vi "Demo Math Tester.vi"() -> ()   [LabVIEW 2014]
uses:
  <vilib>/Utility/miscctls.llb/LVRowAndColumnTypeDef.ctl
  <vilib>/Utility/miscctls.llb/LVPointTypeDef.ctl
  MathLoop/TypeDefs/ParsedExpression.ctl
  MathLoop/TypeDefs/typeMed.ctl
  MathLoop/TypeDefs/Conf. Gral.ctl
  APIs/Data Queue/Acquisition Data 1 Sample Cluster.ctl
  <vilib>/Analysis/2dsp.llb/Real FFT.vi
  <vilib>/Analysis/2dsp.llb/Inverse Real FFT.vi
  <vilib>/Analysis/2dsp.llb/Inverse Complex FFT.vi
  MathLoop/TypeDefs/Globals.vi
  APIs/Message Queue/Enqueue Message (Single).vi
  <vilib>/Utility/file.llb/Write To Spreadsheet File (string).vi
  APIs/Data Queue/WINFAS 2 Data Queue.lvlib
  APIs/Message Queue/WINFAS 2 Message Queue.lvlib
  MathLoop/MathLoop.lvlib
  <vilib>/Analysis/NI_AALPro.lvlib
panel:
  in  "Config:Mapp":bool
  out "MedPath":string
  out "TransPath":string caption="Último Cálculo:"
  in  "error in (no error)":errorcluster
  out "Time":dbl=0.7666387252129425 format="%#_6fseg"
  out "LAST":string="28/08/2015 08:45:35 a.m." caption="Último Cálculo:"
  in  "Medicion (Solo P/ Resultado Post-Proceso):":i32=1 min=0 max=0 format="M%.0f"
  out "Medición":string[][](table)
  out "Curva de Engranes":dbl[][](graph)
  out "Transductores":string[][](table)
  in  "Config Aux & Med":bool
  in  "Save Cfg":bool
  in  "Start":bool
  in  "Open Cfg":bool
  in  "New Cfg":bool
  # "Configuración"
  # "Curva de Engrane"
  # "Archivos:"
  # "Tabla de Transductores"
  # "Proceso de medición"
  # "Último Cálculo:"
  # "Tiempo de Cálculo:"
  # "Medición"
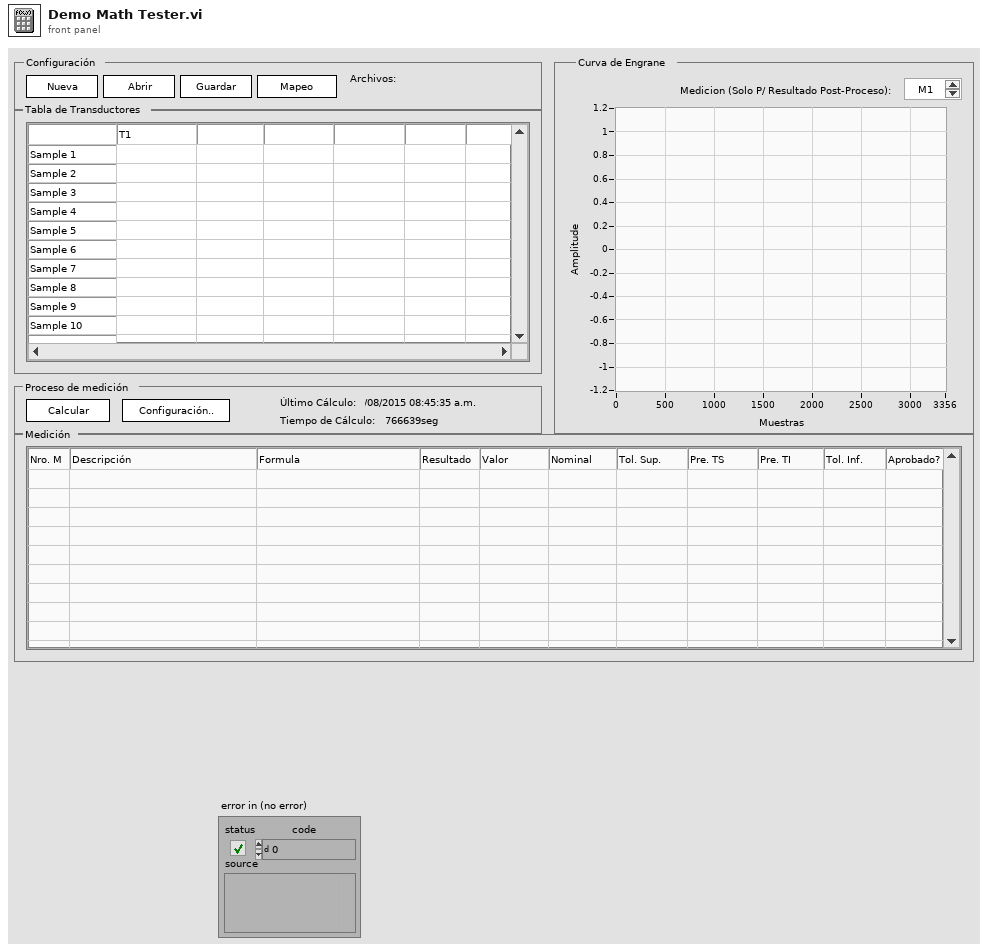
[diagram p1: front panel]
types:
  T1 = typedef "MathLoop.lvlib/ParsedExpression.ctl" = cluster{"RPN ":string[], "Constantes":sgl[], "Variables":string[], "Formula":string, "Tipo de Med":T2, "Med?":bool, "Descripción":string, "Nominal":sgl, "Tol Sup":sgl, "Pre TS":sgl, "Pre TI":sgl, "Tol Inf":sgl}
  T2 = typedef "MathLoop.lvlib/typeMed.ctl" = string
  T3 = typedef "MathLoop.lvlib/Conf. Gral.ctl" = cluster{"Engranometro":cluster{"Cant. Dientes x pieza":i32, "Nro. Dientes (Frp)":i32, "Armonicas":i32}}
  T4 = cluster{"Variable Data Out":cluster{"Kcte":sgl[], "Dcte":sgl[], "Aux":sgl[][], "Transductores":sgl[][]}, "Array":sgl[], T1[], "Array Med":sgl[][], "Conf. General":T3}
  T5 = typedef "LVPointTypeDef.ctl" = cluster{"Horizontal":i16, "Vertical":i16}
  T6 = typedef "LVRowAndColumnTypeDef.ctl" = cluster{"Row":i32, "Column":i32}
  T7 = enum32{"invalid app kind", "Development System", "Run Time System", "Student Edition", "Embedded LabVIEW", "Evaluation", "Custom"}
  T8 = typedef "WINFAS 2 Message Queue.lvlib/All Message Queues.ctl" = cluster{"CORE":refnum<queue>, "Event UI":refnum<queue>, "Display UI":refnum<queue>, "MATH":refnum<queue>, "SEQ":refnum<queue>, "DB":refnum<queue>, "ERR":refnum<queue>, "HAL":refnum<queue>, "HWSync1":refnum<queue>, "HWSync2":refnum<queue>, "HWSync3":refnum<queue>, "HWSync4":refnum<queue>, "HWSync5":refnum<queue>, "HWAsync1":refnum<queue>, "HWAsync2":refnum<queue>, "HWAsync3":refnum<queue>, "HWAsync4":refnum<queue>, "HWAsync5":refnum<queue>, "HWAsync6":refnum<queue>, "HWAsync7":refnum<queue>, "HWAsync8":refnum<queue>, "HWAsync9":refnum<queue>, "HWAsync10":refnum<queue>}
  T9 = typedef "WINFAS 2 Data Queue.lvlib/All Data Queues Cluster.ctl" = cluster{"Queues":cluster{"ACQ HWSync1":refnum<queue>, "ACQ HWSync2":refnum<queue>, "ACQ HWSync3":refnum<queue>, "ACQ HWSync4":refnum<queue>, "ACQ HWSync5":refnum<queue>}, "Notifiers":cluster{"Control":cluster{"CTRL HWSync1":refnum<notifier>, "CTRL HWSync2":refnum<notifier>, "CTRL HWSync3":refnum<notifier>, "CTRL HWSync4":refnum<notifier>, "CTRL HWSync5":refnum<notifier>}, "Acquisition":cluster{"ACQ HWSync1":refnum<notifier>, "ACQ HWSync2":refnum<notifier>, "ACQ HWSync3":refnum<notifier>, "ACQ HWSync4":refnum<notifier>, "ACQ HWSync5":refnum<notifier>}, "Async":cluster{"ACQ HWAsync1":refnum<notifier>, "ACQ HWAsync2":refnum<notifier>, "ACQ HWAsync3":refnum<notifier>, "ACQ HWAsync4":refnum<notifier>, "ACQ HWAsync5":refnum<notifier>, "ACQ HWAsync6":refnum<notifier>, "ACQ HWAsync7":refnum<notifier>, "ACQ HWAsync8":refnum<notifier>, "ACQ HWAsync9":refnum<notifier>, "ACQ HWAsync10":refnum<notifier>}}}
  T10 = cluster{"Array Parsed Expression":T1[], "Nominal":sgl[], "Total Inferior":sgl[], "Total Superior":sgl[], "Pre Total Inferior":sgl[], "Pre Total Superior":sgl[], "Descripción":string[]}
  T11 = typedef "WINFAS 2 Data Queue.lvlib/Acquisition Data 1 Sample Cluster.ctl" = cluster{"TDX":sgl[], "Encoder":sgl}
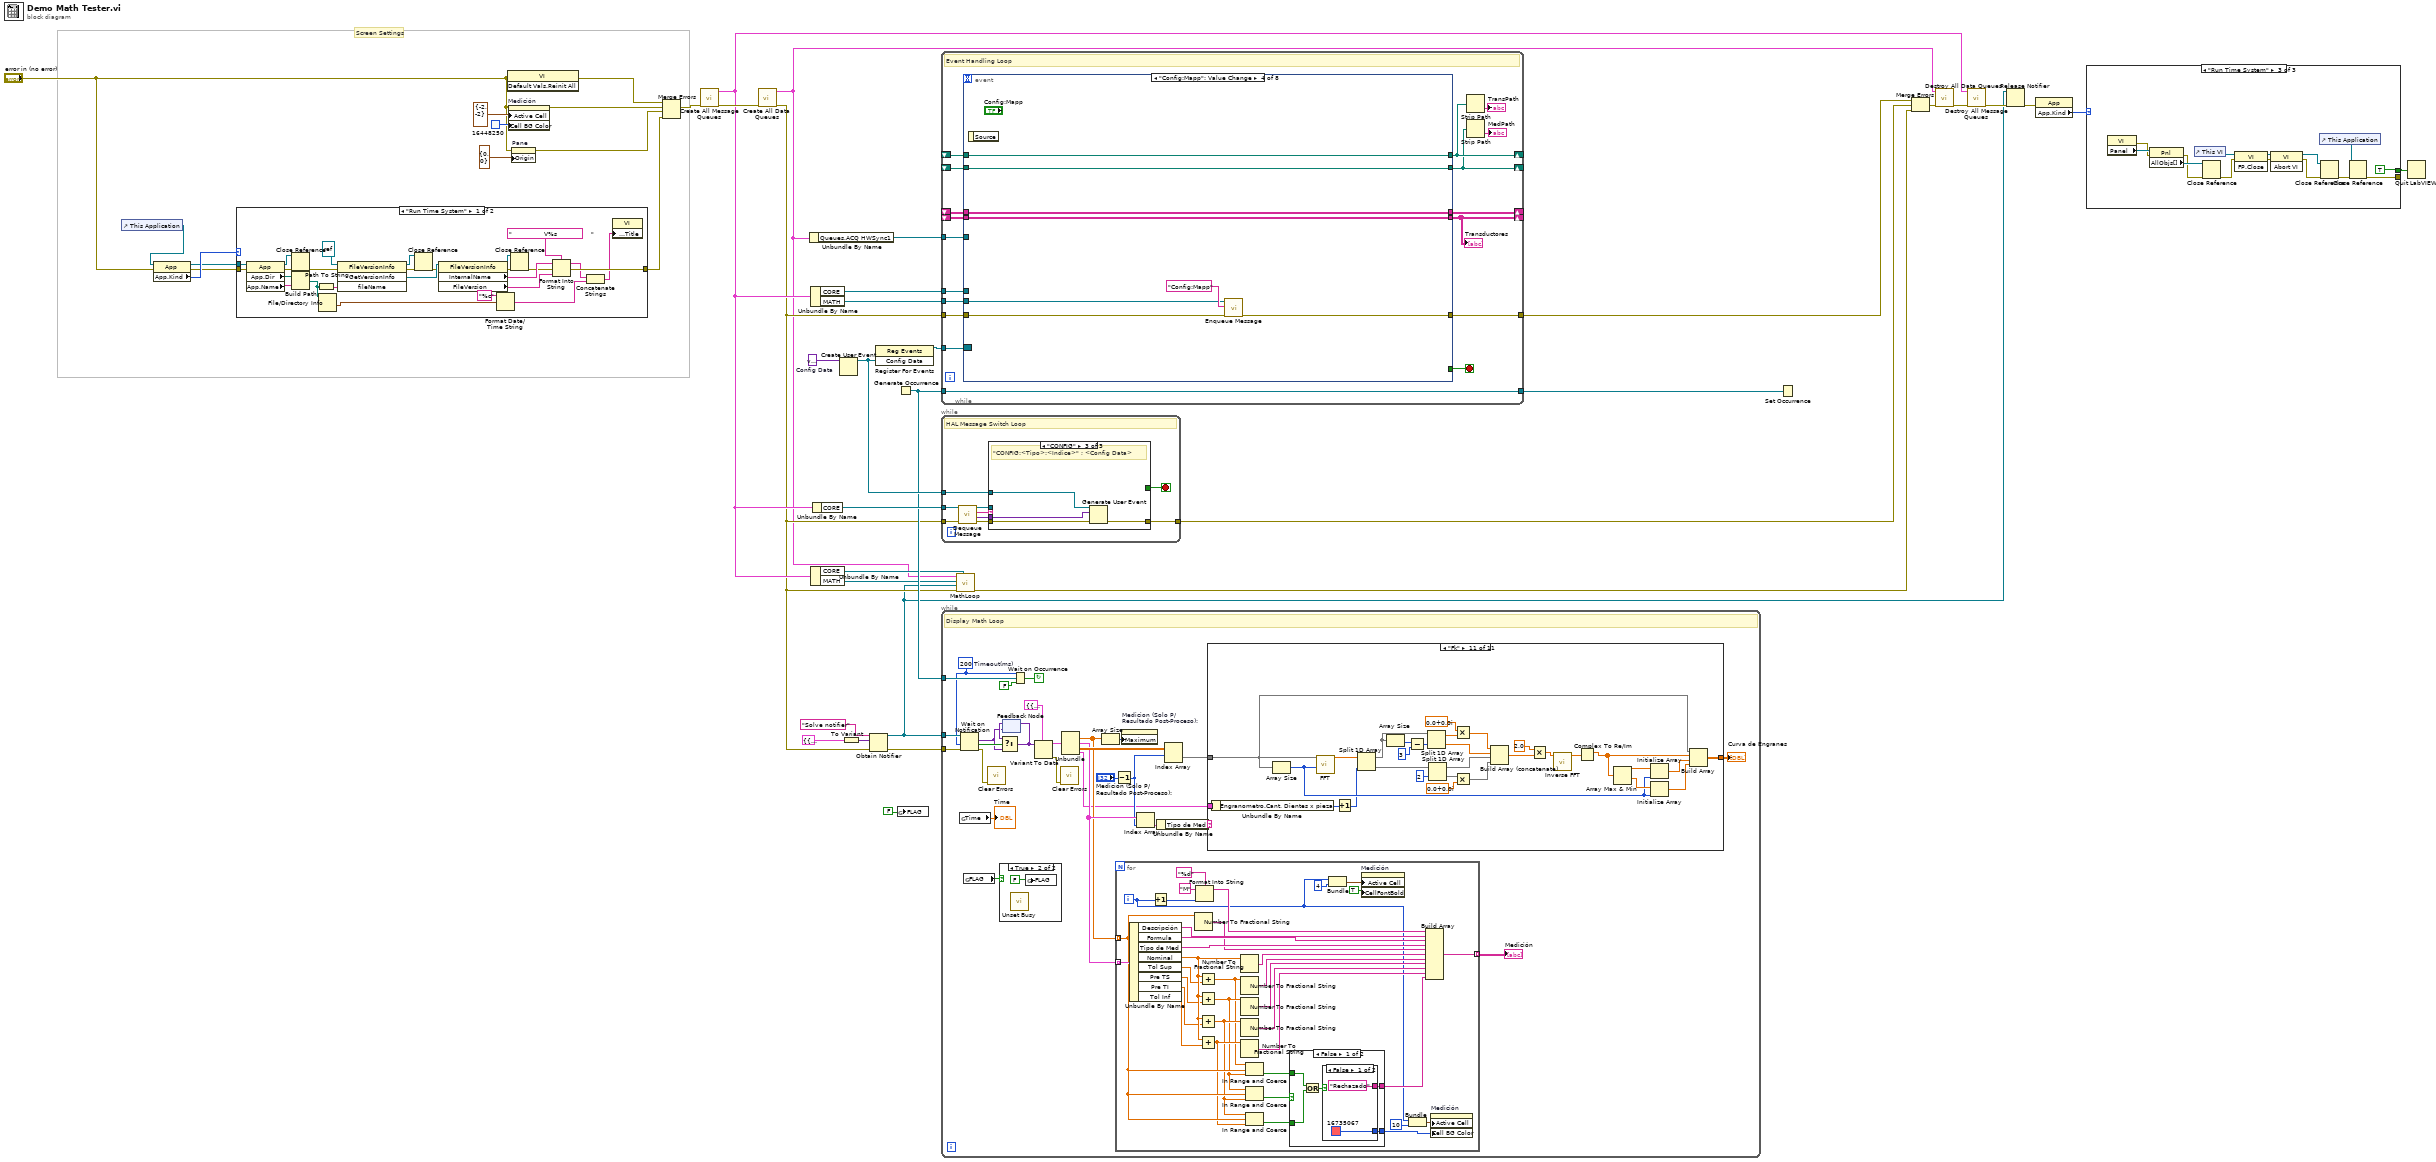
[diagram p0: block diagram]
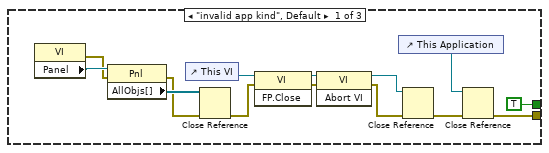
[diagram p3: hidden frame]
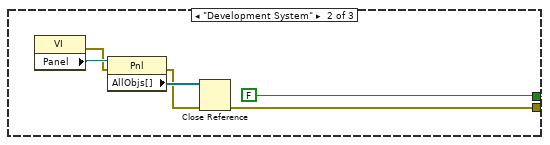
[diagram p4: hidden frame]
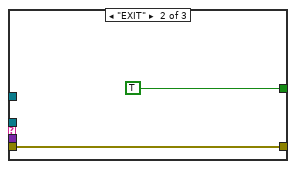
[diagram p6: hidden frame]
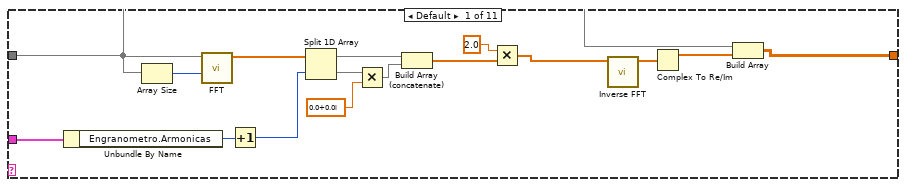
[diagram p8: hidden frame]
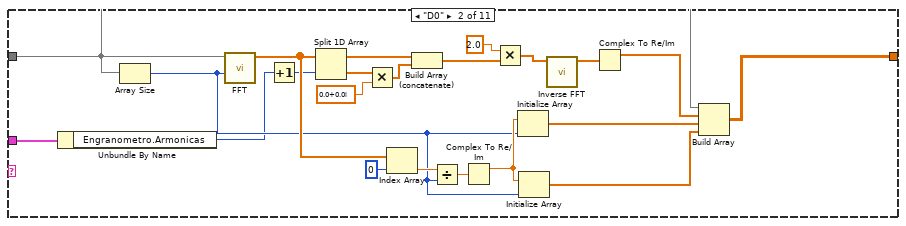
[diagram p9: hidden frame]
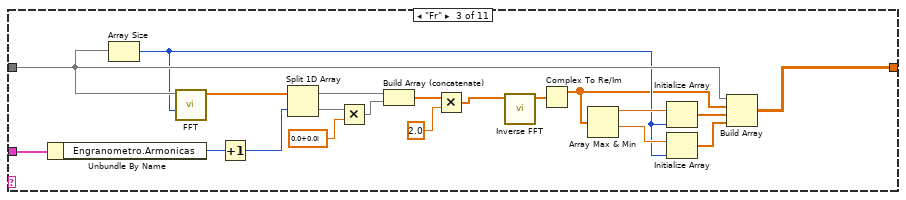
[diagram p10: hidden frame]
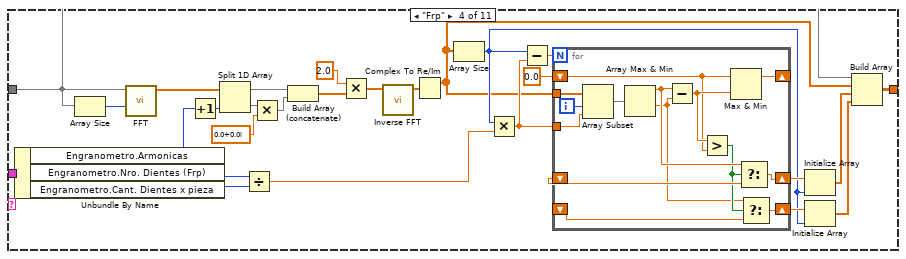
[diagram p11: hidden frame]
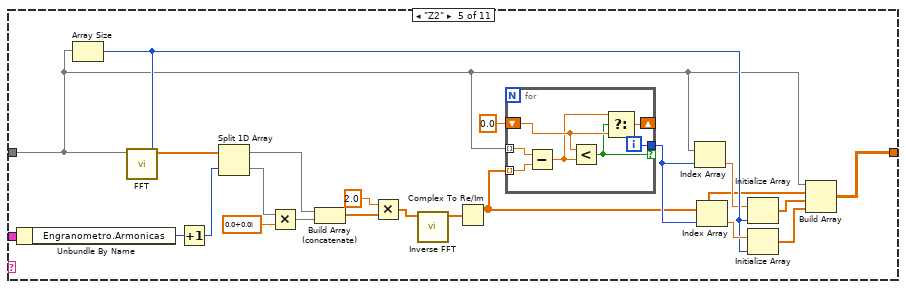
[diagram p12: hidden frame]
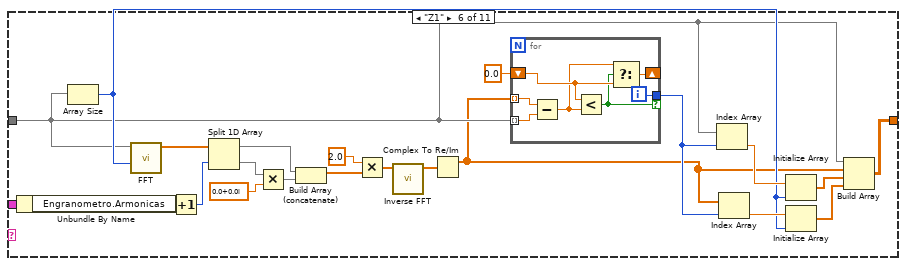
[diagram p13: hidden frame]
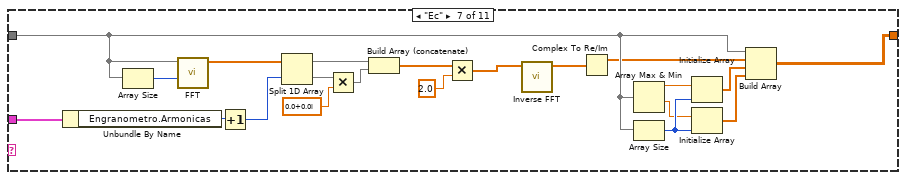
[diagram p14: hidden frame]
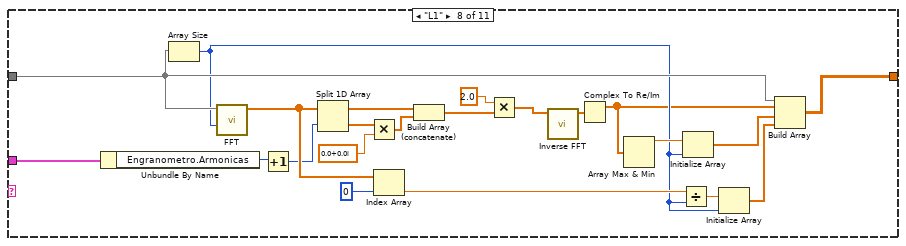
[diagram p15: hidden frame]
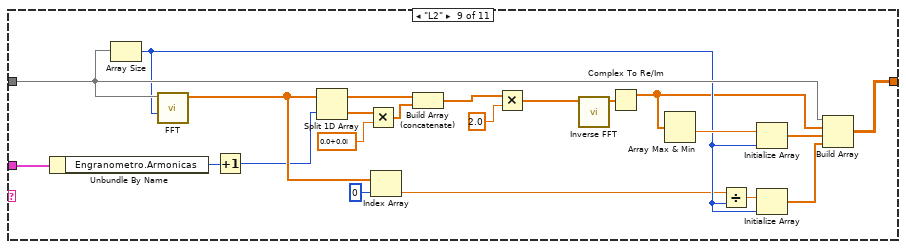
[diagram p16: hidden frame]
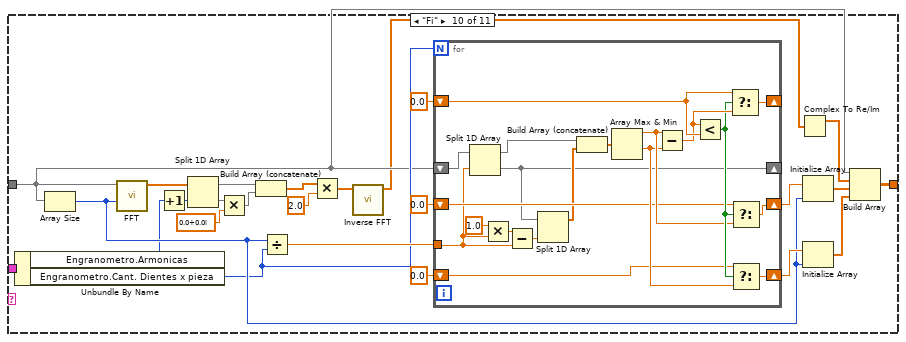
[diagram p17: hidden frame]
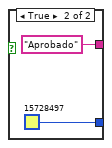
[diagram p18: hidden frame]
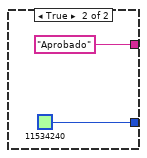
[diagram p19: hidden frame]
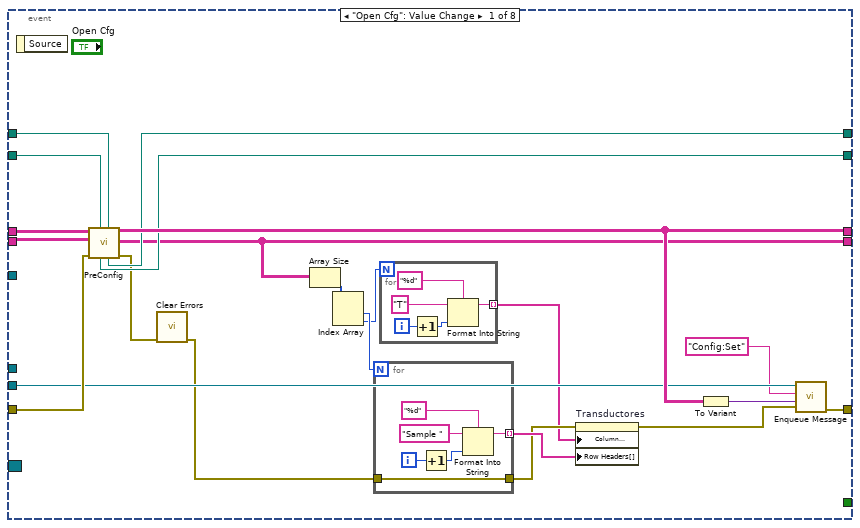
[diagram p20: hidden frame]
diagram:
  w31 = variant  # Config Data
  # "Screen Settings"
  n1 = control-ref of="This Application"() -> (w3:refnum<vi>)
  n2 = property class="App"(reference=w3, error in="error in (no error)") -> (reference out=w4:refnum<vi>, error out=w5:errorcluster, "App.Kind"=w6:T7)
  n3 = case shown="\"Run Time System\"" w6 {
    tunnel: w5 -> [w67 w69]
    tunnel: w4 -> [w68 _]
    tunnel: [w60 w69] -> w1
    frame "Run Time System" {
      n4 = property class="App"(reference=w68, error in=w67) -> (reference out=w48:refnum<vi>, error out=w65:errorcluster, "App.Dir"=w55:path, "App.Name"=w54:string)
      n5 = Close Reference(reference=w48, error in (no error)=w65) -> (error out=w64:errorcluster)
      n6 = Build Path(base path=w55, name or relative path=w54) -> (appended path=w52:path)
      n7 = Path To String(path=w52) -> (string=w66:string)
      n8 = File/Directory Info(path=w52) -> (last mod=w47:timestamp)  [unwired: 1 in, 6 out]
      n9 = invoke class="FileVersionInfo" method="GetVersionInfo"(reference=refnum<k24> refnum, error in=w64, "fileName"=w66) -> (reference out=w50:refnum<k24>, error out=w51:errorcluster, "GetVersionInfo"=w63:refnum<k24>)  [unwired: 1 in, 1 out]
      n10 = Close Reference(reference=w50, error in (no error)=w51) -> (error out=w49:errorcluster)
      n11 = property class="FileVersionInfo"(reference=w63, error in=w49) -> (reference out=w56:refnum<k24>, error out=w58:errorcluster, "InternalName"=w62:string, "FileVersion"=w61:string)
      n12 = Format Date/Time String(time format string (%c)="%c", seconds (now)=w47) -> (date/time string=w45:string)  [unwired: 1 in]
      n13 = Close Reference(reference=w56, error in (no error)=w58) -> (error out=w57:errorcluster)
      n14 = Format Into String(format string="                V%s                 ", initial string=w62, error in=w57, w61) -> (resulting string=w44:string, error out=w60:errorcluster)
      n15 = Concatenate Strings(w44, w45) -> (w43:string)
      n16 = property class="VI"("Front Panel.Title"=w43) -> ()  [unwired: 2 in, 2 out]
    }
    frame "Development System", Default {
    }
  }
  n17 = invoke on="Invoke Node" class="VI" method="Default Vals.Reinit All"(error in="error in (no error)") -> (error out=w18:errorcluster)  [unwired: 2 in, 2 out]
  n18 = property on="Medición" class="Tbl (strict)"(error in="error in (no error)", "Active Cell"=T6 {"Row"=-2, "Column"=-2} ("Active Cell:Active Cell"), "Cell BG Color"=u32 16448250) -> (error out=w19:errorcluster)  [unwired: 1 in, 1 out]
  n19 = property on="Pane" class="Pane"(error in="error in (no error)", "Origin"=T5 {"Horizontal"=0, "Vertical"=0}) -> (error out=w15:errorcluster)  [unwired: 1 in, 1 out]
  n20 = Merge Errors(w18, w19, w15, w1) -> (w20:errorcluster)
  n21 = call "Create All Message Queues.vi"("error in (no error)"=w20) -> ("error out"=w41:errorcluster, "Message Queues Out"=w33:T8)  [unwired: 9 in]
  n22 = call "Create All Data Queues.vi"("Error In"=w41) -> ("Error Out"=w11:errorcluster, "WINFAS 2 Data Queue.lvlib:All Data Queues Cluster"=w9:T9)  [unwired: 9 in]
  n23 = Unbundle By Name(w9) -> ("Queues.ACQ HWSync1"=w37:refnum<queue>)
  n24 = Unbundle By Name(w33) -> ("CORE"=w28:refnum<queue>, "MATH"=w34:refnum<queue>)
  n25 = Unbundle By Name(w33) -> ("CORE"=w10:refnum<queue>, "MATH"=w8:refnum<queue>)
  n26 = Unbundle By Name(w33) -> ("CORE"=w32:refnum<queue>)
  n27 = Create User Event(user event datatype=w31) -> (user event=w30:refnum<user-event>)  [unwired: 1 in, 1 out]
  n28 = To Variant(anything=T4 {"Variable Data Out"={"Kcte"=[], "Dcte"=[], "Aux"=[], "Transductores"=[]}, "Array"=[], [], "Array Med"=[], "Conf. General"={"Engranometro"={"Cant. Dientes x pieza"=0, "Nro. Dientes (Frp)"=0, "Armonicas"=0}}} ("output cluster")) -> (Variant=w39:variant)
  n29 = Obtain Notifier(name (unnamed)="Solve notifier", notification data type=w39) -> (notifier out=w7:refnum<notifier>)  [unwired: 2 in, 2 out]
  n30 = register-events(w30) -> (reference out=w29:refnum<event-registration>)  [unwired: 2 in, 1 out]
  n31 = Generate Occurrence() -> (w26:refnum<k4>)
  n32 = global write "Globals.vi" "FLAG"(FALSE ("FLAG")) -> ()
  n33 = while {
    tunnel: w37 -> [w87]
    tunnel: [w86] -> w35
    tunnel: w34 -> [w85]
    tunnel: w11 -> [w84]
    shift-right: [w81] -> _
    shift-left: _ -> [w79]
    shift-right: [w82] -> _
    shift-left: _ -> [w80]
    tunnel: w29 -> [w78]
    tunnel: w28 -> [w77]
    tunnel: [w76] -> w27
    tunnel: w26 -> [w76]
    shift-right: [w71] -> _
    shift-left: _ -> [w75]
    shift-right: [w70] -> _
    shift-left: _ -> [w74]
    stop <- w83 stop-if-true
    # "Event Handling Loop"
    n34 = event shown="[3] \"Config:Mapp\": Value Change" {
      selector: w78 -> [_ _ _ _ _ _ _ _]
      dyn-events: _ -> [_ _ _ _ _ _ _ _]
      timeout: _ -> [_ _ _ _ _ _ _ _]
      tunnel: w87 -> [_ _ _ _ _ _ w204 _]
      tunnel: [w108 w124 w143 w147 _ w183 w206 w226] -> w86
      tunnel: w85 -> [w105 _ _ w148 _ w185 w207 w231]
      tunnel: w84 -> [w109 w127 w143 w149 _ w184 w192 w232]
      tunnel: [_ _ _ _ _ _ _ TRUE ("EXIT")] -> w83
      tunnel: [w107 w125 w132 w154 w163 w181 w205 w229] -> w82
      tunnel: [w91 w123 w142 w153 w162 w182 w202 w230] -> w81
      tunnel: w80 -> [w103 _ w132 w154 w161 w181 w205 w229]
      tunnel: w79 -> [w102 w123 w142 w153 w160 w182 w202 w230]
      tunnel: w77 -> [_ _ _ _ _ _ _ w225]
      tunnel: [w101 w122 w131 w152 path "" ("Ruta de Transductores Out") w178 w194 w222] -> w71
      tunnel: [w100 w121 w130 w151 path "" ("Ruta de Mediciones Out") w177 w193 w221] -> w70
      tunnel: w75 -> [w99 w122 w131 w152 _ w178 w194 w222]
      tunnel: w74 -> [w98 w121 w130 w151 _ w177 w193 w221]
      event "Open Cfg": Value Change {
        n35 = event-data() -> ()  [unwired: 1 in, 1 out]
        n36 = call "PreConfig.vi"("Ruta de Transductores in"=w99, "Ruta de Mediciones in"=w98, "error in (no error)"=w109, "Transductores"=w102, "Medidas"=w103) -> ("error out"=w97:errorcluster, "Transductores"=w91:string[][], "Mediciones"=w107:string[][], "Ruta de Transductores Out"=w101:path, "Ruta de Mediciones Out"=w100:path)  [unwired: 2 in]
        n37 = call <vilib>:"Clear Errors.vi"("error in (no error)"=w97) -> ("error out"=w93:errorcluster)  [unwired: 5 in, 1 out]
        n38 = Array Size(array=w91) -> (size(s)=w90:i32[])
        n39 = Index Array(array=w90) -> (element #1=w89:i32, element #2=w88:i32)  [unwired: 2 in]
        n40 = for {
          N: w89 -> [_]
          tunnel: [w120] -> w96 mode=indexing
          tunnel: [w115] -> w95
          tunnel: w93 -> [w115]
          i -> [w117]
          n41 = Increment(x=w117) -> (x+1=w116:i32)
          n42 = Format Into String(format string="%d", initial string="Sample ", w116) -> (resulting string=w120:string)  [unwired: 1 in, 1 out]
        }
        n43 = for {
          N: w88 -> [_]
          tunnel: [w114] -> w94 mode=indexing
          i -> [w111]
          n44 = Increment(x=w111) -> (x+1=w110:i32)
          n45 = Format Into String(format string="%d", initial string="T", w110) -> (resulting string=w114:string)  [unwired: 1 in, 1 out]
        }
        n46 = property on="Transductores" class="Tbl (strict)"(error in=w95, "Column Headers[]"=w94, "Row Headers[]"=w96) -> (error out=w92:errorcluster)  [unwired: 1 in, 1 out]
        n47 = To Variant(anything=w107) -> (Variant=w106:variant)
        n48 = call-poly "Enqueue Message.vi"("error in (no error)"=w92, "Message Data"=w106, "Message"="Config:Set", "Message Queue"=w105) -> ("error out"=w108:errorcluster)  [unwired: 6 in, 1 out]
      }
      event User Event {
        n49 = event-data() -> ("Config Data"=w128:variant)  [unwired: 1 in]
        n50 = Variant To Data(error in=w127, type=string[][] [], Variant=w128) -> (data=w125:string[][], error out=w124:errorcluster)
      }
      event "Save Cfg": Value Change {
        n51 = event-data() -> ()  [unwired: 1 in, 1 out]
        n52 = call <vilib>:"Application Directory.vi"() -> ("Application Directory"=w139:path)
        n53 = Build Path(base path=w139, name or relative path="Resources") -> (appended path=w141:path)
        n54 = call "File Dialog"("start path"=w141, "prompt"="Seleccione el archivo de Configuración (.csv)", "button label"="Guardar Configuración", "pattern (all files)"="*.csv", "pattern label"="Configuración MATH") -> ("selected path"=w133:path, "cancelled"=w129:bool, "error out"=w138:errorcluster)  [unwired: 7 in, 1 out]
        n55 = call <vilib>:"Clear Errors.vi"("error in (no error)"=w138) -> ()  [unwired: 5 in, 2 out]
        n56 = case shown="False" w129 {
          tunnel: w133 -> [w146 _]
          tunnel: w132 -> [w145 _]
          frame False {
            n57 = call-poly <vilib>:"Write To Spreadsheet File.vi"("delimiter (\\t)"="," ("delimiter (\\t)"), "2D data"=w145, "file path (dialog if empty)"=w146) -> ()  [unwired: 5 in, 1 out]
          }
          frame True {
          }
        }
      }
      event "Config:Mapp": Value Change {
        n58 = event-data() -> ()  [unwired: 1 in, 1 out]
        n59 = call-poly "Enqueue Message.vi"("error in (no error)"=w149, "Message"="Config:Mapp", "Message Queue"=w148) -> ("error out"=w147:errorcluster)  [unwired: 7 in, 1 out]
      }
      event "New Cfg": Value Change {
        n60 = event-data() -> ()  [unwired: 1 in, 1 out]
        n61 = Not Equal?(x=w160, y=string[][] [] ("Transductores")) -> (x != y?=w159:bool[][])
        n62 = Empty Array?(array=w159) -> (empty?=w158:bool)
        n63 = Flatten To String(anything=T10 {"Array Parsed Expression"=[], "Nominal"=[], "Total Inferior"=[], "Total Superior"=[], "Pre Total Inferior"=[], "Pre Total Superior"=[], "Descripción"=[]} ("Cluster")) -> (data string=w168:string)  [unwired: 3 in, 2 out]
        n64 = Flatten To String(anything=w161) -> (data string=w169:string)  [unwired: 3 in, 2 out]
        n65 = Not(x=w158) -> (.not. x?=w157:bool)
        n66 = Not Equal?(x=w169, y=w168) -> (x != y?=w165:bool)
        n67 = Or(x=w165, y=w157) -> (x .or. y?=w164:bool)
        n68 = case "Algún Driver cargado?" shown="True" w164 {
          tunnel: [TRUE ("T button?") w173] -> w170
          frame False {
          }
          frame True {
            n69 = Two Button Dialog(message="Desea crear una nueva configuración?\n(Se descargarán todos los Datos cargados)") -> (T button?=w173:bool)  [unwired: 2 in]
          }
        }
        n70 = case shown="True" w170 {
          tunnel: [w175 w176] -> w163
          tunnel: [w174 w176] -> w162
          tunnel: w161 -> [w175 _]
          tunnel: w160 -> [w174 _]
          frame False {
          }
          frame True {
            w176 = string[][] [] ("Transductores")
          }
        }
      }
      event "Config Aux & Med": Value Change {
        n71 = event-data() -> ()  [unwired: 1 in, 1 out]
        n72 = call-poly "Enqueue Message.vi"("error in (no error)"=w184, "Message"="Config", "Message Queue"=w185) -> ("error out"=w183:errorcluster, "dup Message Queue"=w179:refnum<queue>)  [unwired: 7 in]
        n73 = call-poly "Enqueue Message.vi"("Message"="Config:Get", "Message Queue"=w179) -> ()  [unwired: 8 in, 2 out]
      }
      event "Start": Value Change {
        n74 = event-data() -> ()  [unwired: 1 in, 1 out]
        n75 = Get Date/Time In Seconds() -> (seconds since 1Jan1904=w199:timestamp)
        n76 = call <vilib>:"Set Busy.vi"("error in (no error)"=w192) -> ("error out"=w191:errorcluster)  [unwired: 9 in, 1 out]
        n77 = property on="Medición" class="Tbl (strict)"(error in=w191, "Active Cell"=T6 {"Row"=-2, "Column"=-2} ("Active Cell:Active Cell"), "Cell BG Color"=u32 16448250) -> (error out=w195:errorcluster)  [unwired: 1 in, 1 out]
        n78 = Format Date/Time String(seconds (now)=w199) -> (date/time string=→"LAST":string)  [unwired: 2 in]
        n79 = Flush Queue(queue=w204, error in (no error)=w195) -> (queue out=w203:refnum<queue>, error out=w201:errorcluster)  [unwired: 1 out]
        n80 = for {
          tunnel: w203 -> [w216]
          tunnel: w202 -> [w213] mode=indexing
          tunnel: w201 -> [w212]
          tunnel: [w211] -> w200
          n81 = for {
            tunnel: w213 -> [w220] mode=indexing
            tunnel: [w218] -> w217 mode=indexing
            n82 = Fract/Exp String To Number(string=w220, default (0 dbl)=sgl 0.0 ("default (0 DBL)")) -> (number=w218:sgl)  [unwired: 2 in, 1 out]
          }
          n83 = Bundle By Name(cluster=T11 {"TDX"=[0.0, 0.0, 0.0, 0.0, 0.0, 0.0, 0.0, 0.0, 0.0, 0.0, 0.0, 0.0, 0.0, 0.0, 0.0, 0.0, 0.0], "Encoder"=0.0} ("element"), "TDX"=w217) -> (w215:T11)
          n84 = call "Enqueue ACQ Element.vi"("error in (no error)"=w212, "1 Sample"=w215, "ACQ Data Queue in"=w216) -> ("error out"=w211:errorcluster)  [unwired: 7 in, 1 out]
        }
        n85 = flat-sequence {
          tunnel: w200 -> [w209]
          tunnel: [w209] -> w188
          frame #0 {
            n86 = Wait (ms)(milliseconds to wait=u32 50) -> ()  [unwired: 1 out]
          }
        }
        n87 = property on="Medición" class="Tbl (strict)"(error in=w188, "Active Cell"=T6 {"Row"=-2, "Column"=-2} ("Active Cell:Active Cell"), "Cell BG Color"=u32 16448250) -> (error out=w187:errorcluster)  [unwired: 1 in, 1 out]
        n88 = call-poly "Enqueue Message.vi"("error in (no error)"=w187, "Message"="Solve", "Message Queue"=w207) -> ("error out"=w206:errorcluster)  [unwired: 7 in, 1 out]
      }
      event Panel Close? {
        n89 = event-data() -> ()  [unwired: 1 in, 4 out]
        n90 = call-poly "Enqueue Message.vi"("error in (no error)"=w232, "Message"="EXIT", "Message Queue"=w231) -> ("error out"=w227:errorcluster)  [unwired: 7 in, 1 out]
        n91 = call-poly "Enqueue Message.vi"("error in (no error)"=w227, "Message"="EXIT", "Message Queue"=w225) -> ("error out"=w226:errorcluster)  [unwired: 7 in, 1 out]
        n92 = event-data("Discard?"=TRUE) -> ()  [unwired: 1 in, 1 out]
      }
    }
    "Transductores" <- w81
    n93 = Strip Path(path=w71) -> (name=→"TransPath":string)  [unwired: 1 out]
    n94 = Strip Path(path=w70) -> (name=→"MedPath":string)  [unwired: 1 out]
  }
  n95 = while {
    tunnel: w32 -> [w242]
    tunnel: w11 -> [w241]
    tunnel: [w236] -> w17
    tunnel: w30 -> [w235]
    stop <- w237 stop-if-true
    # "HAL Message Switch Loop"
    n96 = call "Dequeue Message.vi"("error in (no error)"=w241, "Message Queue"=w242) -> ("error out"=w240:errorcluster, "Message Data"=w239:variant, "Message"=w234:string, "dup Message Queue"=w238:refnum<queue>)  [unwired: 6 in]
    n97 = case shown="\"CONFIG\"" w234 {
      tunnel: w240 -> [w243 w244 w247]
      tunnel: w239 -> [_ _ w249]
      tunnel: w238 -> [_ _ _]
      tunnel: [_ TRUE _] -> w237
      tunnel: [w243 w244 w246] -> w236
      tunnel: w235 -> [_ _ w248]
      frame Default {
      }
      frame "EXIT" {
      }
      frame "CONFIG" {
        # "\"CONFIG:<Tipo>:<Indice>\" ; <Config Data>"
        n98 = Generate User Event(user event=w248, event data cluster=w249, error in=w247) -> (error out=w246:errorcluster)  [unwired: 1 in, 1 out]
      }
    }
  }
  n99 = while {
    tunnel: w7 -> [w277]
    tunnel: w11 -> [w276]
    tunnel: w26 -> [w260]
    stop <- w261 continue-if-true
    w259 = 200  # Timeout(ms)
    # "Display Math Loop"
    n100 = global read "Globals.vi" "Time"() -> (→"Time":dbl)
    n101 = Wait on Notification(notifier=w277, timeout in ms (-1)=w259, error in (no error)=w276) -> (notification=w266:variant, timed out?=w267:bool, error out=w264:errorcluster)  [unwired: 1 in, 1 out]
    n102 = global read "Globals.vi" "FLAG"() -> (w253:bool)
    n103 = call <vilib>:"Clear Errors.vi"("error in (no error)"=w264) -> ()  [unwired: 5 in, 2 out]
    n104 = case shown="True" w253 {
      frame False {
      }
      frame True {
        n105 = call <vilib>:"Unset Busy.vi"() -> ()  [unwired: 11 in, 1 out]
        n106 = global write "Globals.vi" "FLAG"(FALSE ("FLAG")) -> ()
      }
    }
    n107 = feedback #1(w266) -> (w268:variant)
    n108 = Select(t=w268, s=w267, f=w266) -> (s? t:f=w265:variant)
    n109 = feedback-in #1(w265) -> ()
    n110 = Wait on Occurrence(1:FALSE ("ignore previous (T)"), 2:w260, 3:w259) -> (0:w261:bool)
    n111 = Variant To Data(type=T4 {"Variable Data Out"={"Kcte"=[], "Dcte"=[], "Aux"=[], "Transductores"=[]}, "Array"=[], [], "Array Med"=[], "Conf. General"={"Engranometro"={"Cant. Dientes x pieza"=0, "Nro. Dientes (Frp)"=0, "Armonicas"=0}}} ("output cluster"), Variant=w265) -> (data=w270:T4, error out=w263:errorcluster)  [unwired: 1 in]
    n112 = call <vilib>:"Clear Errors.vi"("error in (no error)"=w263) -> ()  [unwired: 5 in, 2 out]
    n113 = Unbundle(w270) -> ("Array"=w255:sgl[], w273:T1[], "Array Med"=w275:sgl[][], "Conf. General"=w251:T3)  [unwired: 1 out]
    n114 = Array Size(array=w255) -> (size(s)=w254:i32)
    n115 = Decrement(x="Medicion (Solo P/ Resultado Post-Proceso):") -> (x-1=w256:i32)
    n116 = for {
      tunnel: [w607] -> w269 mode=indexing
      tunnel: w255 -> [w589] mode=indexing
      tunnel: w273 -> [w605] mode=indexing
      i -> [w576]
      n117 = Unbundle By Name(w605) -> ("Descripción"=w598:string, "Formula"=w608:string, "Tipo de Med"=w606:T2, "Nominal"=w597:sgl, "Tol Sup"=w584:sgl, "Pre TS"=w596:sgl, "Pre TI"=w595:sgl, "Tol Inf"=w594:sgl)
      n118 = Increment(x=w576) -> (x+1=w575:i32)
      n119 = Number To Fractional String(number=w589) -> (F-format string=w588:string)  [unwired: 3 in]
      n120 = Format Into String(format string="%d", initial string="M", w575) -> (resulting string=w599:string)  [unwired: 1 in, 1 out]
      n121 = Add(x=w597, y=w584) -> (x+y=w583:sgl)
      n122 = Add(x=w597, y=w596) -> (x+y=w585:sgl)
      n123 = Add(x=w597, y=w595) -> (x+y=w586:sgl)
      n124 = Add(x=w597, y=w594) -> (x+y=w587:sgl)
      n125 = Number To Fractional String(number=w597) -> (F-format string=w604:string)  [unwired: 3 in]
      n126 = Number To Fractional String(number=w583) -> (F-format string=w603:string)  [unwired: 3 in]
      n127 = Number To Fractional String(number=w585) -> (F-format string=w602:string)  [unwired: 3 in]
      n128 = Number To Fractional String(number=w586) -> (F-format string=w601:string)  [unwired: 3 in]
      n129 = Number To Fractional String(number=w587) -> (F-format string=w600:string)  [unwired: 3 in]
      n130 = In Range and Coerce(upper limit=w583, x=w589, lower limit=w585) -> (In Range?=w592:bool)  [unwired: 1 out]
      n131 = In Range and Coerce(upper limit=w585, x=w589, lower limit=w586) -> (In Range?=w593:bool)  [unwired: 1 out]
      n132 = In Range and Coerce(upper limit=w586, x=w589, lower limit=w587) -> (In Range?=w591:bool)  [unwired: 1 out]
      n133 = case shown="False" w593 {
        tunnel: w592 -> [w614 _]
        tunnel: w591 -> [w613 _]
        tunnel: [w612 "Aprobado"] -> w590
        tunnel: [w611 u32 11534240] -> w580
        frame False {
          n134 = Or(x=w614, y=w613) -> (x .or. y?=w615:bool)
          n135 = case shown="False" w615 {
            tunnel: ["Rechazado" "Aprobado"] -> w612
            tunnel: [u32 16735067 u32 15728497] -> w611
            frame False {
            }
            frame True {
            }
          }
        }
        frame True {
        }
      }
      n136 = Bundle(w576, 4) -> (w578:cluster{i32, i32})  [unwired: 1 in]
      n137 = property on="Medición" class="Tbl (strict)"("Active Cell"=w578, "CellFontBold"=TRUE ("Active Cell:Cell Font:Bold")) -> ()  [unwired: 2 in, 2 out]
      n138 = Bundle(w576, 10) -> (w582:cluster{i32, i32})  [unwired: 1 in]
      n139 = Build Array(w599, w598, w608, w606, w588, w604, w603, w602, w601, w600, w590) -> (w607:T2[])
      n140 = property on="Medición" class="Tbl (strict)"("Active Cell"=w582, "Cell BG Color"=w580) -> ()  [unwired: 2 in, 2 out]
    }
    "Medición" <- w269
    n141 = property on="Medicion (Solo P/ Resultado Post-Proceso):" class="DigNum (strict)"("Maximum"=w254) -> ()  [unwired: 2 in, 2 out]
    n142 = Index Array(array=w273, index=w256) -> (element=w272:T1)
    n143 = Unbundle By Name(w272) -> ("Tipo de Med"=w271:T2)
    n144 = Index Array(array=w275, index (row)=w256) -> (element=w274:sgl[])  [unwired: 1 in]
    n145 = case shown="\"Fk\"" w271 {
      tunnel: w274 -> [w288 w308 w325 w350 w387 w414 w444 w470 w492 w511 w555]
      tunnel: [w286 w315 w332 w363 w396 w415 w453 w477 w498 w508 w573] -> w250
      tunnel: w251 -> [w287 w307 w326 w351 w389 w423 w443 w469 w491 w519 w556]
      frame Default {
        n146 = Unbundle By Name(w287) -> ("Engranometro.Armonicas"=w283:i32)
        n147 = Array Size(array=w288) -> (size(s)=w294:i32)
        n148 = call-poly <vilib>:"FFT.vi"("FFT size"=w294, "X"=w288) -> ("FFT {X}"=w293:cdb[])  [unwired: 8 in, 1 out]
        n149 = Increment(x=w283) -> (x+1=w282:i32)
        n150 = Split 1D Array(array=w293, index=w282) -> (first subarray=w292:cdb[], second subarray=w289:cdb[])
        n151 = Multiply(x=w289, y=cdb 0.0+0.0i) -> (x*y=w290:cdb[])
        n152 = Build Array (concatenate)(w292, w290) -> (w280:cdb[])
        n153 = Multiply(x=2.0, y=w280) -> (x*y=w279:cdb[])
        n154 = call-poly <vilib>:"Inverse FFT.vi"("FFT {X}"=w279) -> ("X"=w285:dbl[])  [unwired: 9 in, 1 out]
        n155 = Complex To Re/Im(x + iy=w285) -> (x=w284:dbl[])  [unwired: 1 out]
        n156 = Build Array(w288, w284) -> (w286:dbl[][])
      }
      frame "D0" {
        n157 = Unbundle By Name(w307) -> ("Engranometro.Armonicas"=w299:i32)
        n158 = Array Size(array=w308) -> (size(s)=w302:i32)
        n159 = call-poly <vilib>:"FFT.vi"("FFT size"=w302, "X"=w308) -> ("FFT {X}"=w305:cdb[])  [unwired: 8 in, 1 out]
        n160 = Increment(x=w299) -> (x+1=w298:i32)
        n161 = Split 1D Array(array=w305, index=w298) -> (first subarray=w309:cdb[], second subarray=w312:cdb[])
        n162 = Multiply(x=w312, y=cdb 0.0+0.0i) -> (x*y=w311:cdb[])
        n163 = Index Array(array=w305, index=0) -> (element=w303:cdb)
        n164 = Build Array (concatenate)(w309, w311) -> (w296:cdb[])
        n165 = Divide(x=w303, y=w302) -> (x/y=w304:cdb)
        n166 = Complex To Re/Im(x + iy=w304) -> (x=w306:dbl)  [unwired: 1 out]
        n167 = Multiply(x=2.0, y=w296) -> (x*y=w295:cdb[])
        n168 = Initialize Array(w306, w302) -> (w314:dbl[])
        n169 = Initialize Array(w306, w302) -> (w313:dbl[])
        n170 = call-poly <vilib>:"Inverse FFT.vi"("FFT {X}"=w295) -> ("X"=w301:cdb[])  [unwired: 9 in, 1 out]
        n171 = Complex To Re/Im(x + iy=w301) -> (x=w300:dbl[])  [unwired: 1 out]
        n172 = Build Array(w308, w300, w314, w313) -> (w315:dbl[][])
      }
      frame "Fr" {
        n173 = Unbundle By Name(w326) -> ("Engranometro.Armonicas"=w321:i32)
        n174 = Array Size(array=w325) -> (size(s)=w324:i32)
        n175 = call-poly <vilib>:"FFT.vi"("FFT size"=w324, "X"=w325) -> ("FFT {X}"=w327:cdb[])  [unwired: 8 in, 1 out]
        n176 = Increment(x=w321) -> (x+1=w320:i32)
        n177 = Split 1D Array(array=w327, index=w320) -> (first subarray=w328:cdb[], second subarray=w331:cdb[])
        n178 = Multiply(x=w331, y=cdb 0.0+0.0i) -> (x*y=w330:cdb[])
        n179 = Build Array (concatenate)(w328, w330) -> (w318:cdb[])
        n180 = Multiply(x=w318, y=2.0 ("x")) -> (x*y=w317:cdb[])
        n181 = call-poly <vilib>:"Inverse FFT.vi"("FFT {X}"=w317) -> ("X"=w323:cdb[])  [unwired: 9 in, 1 out]
        n182 = Complex To Re/Im(x + iy=w323) -> (x=w322:dbl[])  [unwired: 1 out]
        n183 = Array Max & Min(array=w322) -> (max value=w334:dbl, min value=w333:dbl)  [unwired: 2 out]
        n184 = Initialize Array(w334, w324) -> (w336:dbl[])
        n185 = Initialize Array(w333, w324) -> (w335:dbl[])
        n186 = Build Array(w325, w322, w336, w335) -> (w332:dbl[][])
      }
      frame "Frp" {
        n187 = Unbundle By Name(w351) -> ("Engranometro.Armonicas"=w340:i32, "Engranometro.Nro. Dientes (Frp)"=w354:i32, "Engranometro.Cant. Dientes x pieza"=w353:i32)
        n188 = Array Size(array=w350) -> (size(s)=w362:i32)
        n189 = call-poly <vilib>:"FFT.vi"("FFT size"=w362, "X"=w350) -> ("FFT {X}"=w361:cdb[])  [unwired: 8 in, 1 out]
        n190 = Increment(x=w340) -> (x+1=w341:i32)
        n191 = Split 1D Array(array=w361, index=w341) -> (first subarray=w360:cdb[], second subarray=w357:cdb[])
        n192 = Divide(x=w354, y=w353) -> (x/y=w352:dbl)
        n193 = Multiply(x=w357, y=cdb 0.0+0.0i) -> (x*y=w358:cdb[])
        n194 = Build Array (concatenate)(w360, w358) -> (w338:cdb[])
        n195 = Multiply(x=2.0, y=w338) -> (x*y=w337:cdb[])
        n196 = call-poly <vilib>:"Inverse FFT.vi"("FFT {X}"=w337) -> ("X"=w343:cdb[])  [unwired: 9 in, 1 out]
        n197 = Complex To Re/Im(x + iy=w343) -> (x=w342:dbl[])  [unwired: 1 out]
        n198 = Array Size(array=w342) -> (size(s)=w346:i32)
        n199 = Multiply(x=w346, y=w352) -> (x*y=w349:dbl)
        n200 = Subtract(x=w346, y=w349) -> (x-y=w355:dbl)
        n201 = for {
          N: w355 -> [_]
          tunnel: w342 -> [w371]
          tunnel: w349 -> [w370]
          shift-right: [w376] -> _
          shift-left: 0.0 ("element") -> [w373]
          shift-right: [w368] -> w348
          shift-left: _ -> [w372]
          shift-right: [w365] -> w347
          shift-left: _ -> [w364]
          i -> [w375]
          n202 = Array Subset(array=w371, index=w375, length=w370) -> (w377:dbl[])
          n203 = Array Max & Min(array=w377) -> (max value=w369:dbl, min value=w366:dbl)  [unwired: 2 out]
          n204 = Subtract(x=w369, y=w366) -> (x-y=w374:dbl)
          n205 = Greater?(x=w374, y=w373) -> (0:w367:bool)
          n206 = Max & Min(x=w373, y=w374) -> (max(x,y)=w376:dbl)  [unwired: 1 out]
          n207 = Select(t=w369, s=w367, f=w372) -> (s? t:f=w368:dbl)
          n208 = Select(t=w366, s=w367, f=w364) -> (s? t:f=w365:dbl)
        }
        n209 = Initialize Array(w348, w346) -> (w345:dbl[])
        n210 = Initialize Array(w347, w346) -> (w344:dbl[])
        n211 = Build Array(w350, w342, w345, w344) -> (w363:dbl[][])
      }
      frame "Z2" {
        n212 = Unbundle By Name(w389) -> ("Engranometro.Armonicas"=w382:i32)
        n213 = Array Size(array=w387) -> (size(s)=w390:i32)
        n214 = call-poly <vilib>:"FFT.vi"("FFT size"=w390, "X"=w387) -> ("FFT {X}"=w391:cdb[])  [unwired: 8 in, 1 out]
        n215 = Increment(x=w382) -> (x+1=w381:i32)
        n216 = Split 1D Array(array=w391, index=w381) -> (first subarray=w392:cdb[], second subarray=w395:cdb[])
        n217 = Multiply(x=w395, y=cdb 0.0+0.0i) -> (x*y=w394:cdb[])
        n218 = Build Array (concatenate)(w392, w394) -> (w379:cdb[])
        n219 = Multiply(x=2.0, y=w379) -> (x*y=w378:cdb[])
        n220 = call-poly <vilib>:"Inverse FFT.vi"("FFT {X}"=w378) -> ("X"=w384:cdb[])  [unwired: 9 in, 1 out]
        n221 = Complex To Re/Im(x + iy=w384) -> (x=w383:dbl[])  [unwired: 1 out]
        n222 = for {
          tunnel: w383 -> [w405] mode=indexing
          tunnel: w387 -> [w406] mode=indexing
          shift-right: [w402] -> _
          shift-left: 0.0 -> [w404]
          tunnel: [w401] -> w386 if=w400
          i -> [w401]
          n223 = Subtract(x=w406, y=w405) -> (x-y=w403:dbl)
          n224 = Less?(x=w404, y=w403) -> (x < y?=w400:bool)
          n225 = Select(t=w403, s=w400, f=w404) -> (s? t:f=w402:dbl)
        }
        n226 = Index Array(array=w387, index=w386) -> (element=w385:sgl)
        n227 = Index Array(array=w383, index=w386) -> (element=w397:dbl)
        n228 = Initialize Array(w385, w390) -> (w399:sgl[])
        n229 = Initialize Array(w397, w390) -> (w398:dbl[])
        n230 = Build Array(w387, w383, w399, w398) -> (w396:dbl[][])
      }
      frame "Z1" {
        n231 = Unbundle By Name(w423) -> ("Engranometro.Armonicas"=w411:i32)
        n232 = Array Size(array=w414) -> (size(s)=w416:i32)
        n233 = call-poly <vilib>:"FFT.vi"("FFT size"=w416, "X"=w414) -> ("FFT {X}"=w424:cdb[])  [unwired: 8 in, 1 out]
        n234 = Increment(x=w411) -> (x+1=w410:i32)
        n235 = Split 1D Array(array=w424, index=w410) -> (first subarray=w425:cdb[], second subarray=w428:cdb[])
        n236 = Multiply(x=w428, y=cdb 0.0+0.0i) -> (x*y=w427:cdb[])
        n237 = Build Array (concatenate)(w425, w427) -> (w408:cdb[])
        n238 = Multiply(x=2.0, y=w408) -> (x*y=w407:cdb[])
        n239 = call-poly <vilib>:"Inverse FFT.vi"("FFT {X}"=w407) -> ("X"=w413:cdb[])  [unwired: 9 in, 1 out]
        n240 = Complex To Re/Im(x + iy=w413) -> (x=w412:dbl[])  [unwired: 1 out]
        n241 = for {
          tunnel: w414 -> [w434] mode=indexing
          tunnel: w412 -> [w435] mode=indexing
          shift-right: [w431] -> _
          shift-left: 0.0 -> [w433]
          tunnel: [w430] -> w421 if=w429
          i -> [w430]
          n242 = Subtract(x=w435, y=w434) -> (x-y=w432:dbl)
          n243 = Less?(x=w433, y=w432) -> (x < y?=w429:bool)
          n244 = Select(t=w432, s=w429, f=w433) -> (s? t:f=w431:dbl)
        }
        n245 = Index Array(array=w414, index=w421) -> (element=w422:sgl)
        n246 = Index Array(array=w412, index=w421) -> (element=w419:dbl)
        n247 = Initialize Array(w422, w416) -> (w417:sgl[])
        n248 = Initialize Array(w419, w416) -> (w418:dbl[])
        n249 = Build Array(w414, w412, w417, w418) -> (w415:dbl[][])
      }
      frame "Ec" {
        n250 = Unbundle By Name(w443) -> ("Engranometro.Armonicas"=w440:i32)
        n251 = Array Size(array=w444) -> (size(s)=w445:i32)
        n252 = call-poly <vilib>:"FFT.vi"("FFT size"=w445, "X"=w444) -> ("FFT {X}"=w446:cdb[])  [unwired: 8 in, 1 out]
        n253 = Increment(x=w440) -> (x+1=w439:i32)
        n254 = Split 1D Array(array=w446, index=w439) -> (first subarray=w447:cdb[], second subarray=w450:cdb[])
        n255 = Multiply(x=w450, y=cdb 0.0+0.0i) -> (x*y=w449:cdb[])
        n256 = Build Array (concatenate)(w447, w449) -> (w437:cdb[])
        n257 = Multiply(x=w437, y=2.0 ("x")) -> (x*y=w436:cdb[])
        n258 = call-poly <vilib>:"Inverse FFT.vi"("FFT {X}"=w436) -> ("X"=w442:cdb[])  [unwired: 9 in, 1 out]
        n259 = Complex To Re/Im(x + iy=w442) -> (x=w441:dbl[])  [unwired: 1 out]
        n260 = Array Max & Min(array=w444) -> (max value=w452:sgl, min value=w451:sgl)  [unwired: 2 out]
        n261 = Array Size(array=w444) -> (size(s)=w454:i32)
        n262 = Initialize Array(w452, w454) -> (w456:sgl[])
        n263 = Initialize Array(w451, w454) -> (w455:sgl[])
        n264 = Build Array(w444, w441, w456, w455) -> (w453:dbl[][])
      }
      frame "L1" {
        n265 = Unbundle By Name(w469) -> ("Engranometro.Armonicas"=w461:i32)
        n266 = Array Size(array=w470) -> (size(s)=w465:i32)
        n267 = call-poly <vilib>:"FFT.vi"("FFT size"=w465, "X"=w470) -> ("FFT {X}"=w468:cdb[])  [unwired: 8 in, 1 out]
        n268 = Increment(x=w461) -> (x+1=w460:i32)
        n269 = Split 1D Array(array=w468, index=w460) -> (first subarray=w471:cdb[], second subarray=w474:cdb[])
        n270 = Multiply(x=w474, y=cdb 0.0+0.0i) -> (x*y=w473:cdb[])
        n271 = Index Array(array=w468, index=0) -> (element=w467:cdb)
        n272 = Build Array (concatenate)(w471, w473) -> (w458:cdb[])
        n273 = Multiply(x=2.0, y=w458) -> (x*y=w457:cdb[])
        n274 = call-poly <vilib>:"Inverse FFT.vi"("FFT {X}"=w457) -> ("X"=w463:cdb[])  [unwired: 9 in, 1 out]
        n275 = Complex To Re/Im(x + iy=w463) -> (x=w462:dbl[])  [unwired: 1 out]
        n276 = Array Max & Min(array=w462) -> (max value=w475:dbl)  [unwired: 3 out]
        n277 = Divide(x=w467, y=w465) -> (x/y=w466:cdb)
        n278 = Initialize Array(w475, w465) -> (w478:dbl[])
        n279 = Initialize Array(w466, w465) -> (w464:cdb[])
        n280 = Build Array(w470, w462, w478, w464) -> (w477:cdb[][])
      }
      frame "L2" {
        n281 = Unbundle By Name(w491) -> ("Engranometro.Armonicas"=w483:i32)
        n282 = Array Size(array=w492) -> (size(s)=w487:i32)
        n283 = call-poly <vilib>:"FFT.vi"("FFT size"=w487, "X"=w492) -> ("FFT {X}"=w490:cdb[])  [unwired: 8 in, 1 out]
        n284 = Increment(x=w483) -> (x+1=w482:i32)
        n285 = Split 1D Array(array=w490, index=w482) -> (first subarray=w493:cdb[], second subarray=w496:cdb[])
        n286 = Multiply(x=w496, y=cdb 0.0+0.0i) -> (x*y=w495:cdb[])
        n287 = Index Array(array=w490, index=0) -> (element=w486:cdb)
        n288 = Build Array (concatenate)(w493, w495) -> (w480:cdb[])
        n289 = Multiply(x=w480, y=2.0 ("x")) -> (x*y=w479:cdb[])
        n290 = call-poly <vilib>:"Inverse FFT.vi"("FFT {X}"=w479) -> ("X"=w485:cdb[])  [unwired: 9 in, 1 out]
        n291 = Complex To Re/Im(x + iy=w485) -> (x=w484:dbl[])  [unwired: 1 out]
        n292 = Array Max & Min(array=w484) -> (min value=w497:dbl)  [unwired: 3 out]
        n293 = Divide(x=w486, y=w487) -> (x/y=w489:cdb)
        n294 = Initialize Array(w497, w487) -> (w500:dbl[])
        n295 = Initialize Array(w489, w487) -> (w488:cdb[])
        n296 = Build Array(w492, w484, w500, w488) -> (w498:cdb[][])
      }
      frame "Fi" {
        n297 = Unbundle By Name(w519) -> ("Engranometro.Armonicas"=w504:i32, "Engranometro.Cant. Dientes x pieza"=w512:i32)
        n298 = Array Size(array=w511) -> (size(s)=w513:i32)
        n299 = call-poly <vilib>:"FFT.vi"("FFT size"=w513, "X"=w511) -> ("FFT {X}"=w525:cdb[])  [unwired: 8 in, 1 out]
        n300 = Increment(x=w504) -> (x+1=w505:i32)
        n301 = Split 1D Array(array=w525, index=w505) -> (first subarray=w524:cdb[], second subarray=w521:cdb[])
        n302 = Multiply(x=w521, y=cdb 0.0+0.0i) -> (x*y=w522:cdb[])
        n303 = Build Array (concatenate)(w524, w522) -> (w502:cdb[])
        n304 = Divide(x=w513, y=w512) -> (x/y=w520:dbl)
        n305 = Multiply(x=w502, y=2.0 ("x")) -> (x*y=w501:cdb[])
        n306 = call-poly <vilib>:"Inverse FFT.vi"("FFT {X}"=w501) -> ("X"=w507:cdb[])  [unwired: 9 in, 1 out]
        n307 = for {
          N: w512 -> [_]
          shift-right: [w543] -> w514
          shift-left: sgl 0.0 -> [w534]
          shift-right: [w526] -> _
          shift-left: w511 -> [w544]
          tunnel: w520 -> [w530]
          shift-right: [w542] -> w515
          shift-left: sgl 0.0 -> [w535]
          shift-right: [w541] -> _
          shift-left: sgl 0.0 -> [w540]
          n308 = Split 1D Array(array=w544, index=w530) -> (first subarray=w528:sgl[], second subarray=w526:sgl[])
          n309 = Multiply(x=1.0, y=w530) -> (x*y=w532:dbl)
          n310 = Subtract(x=w532, y=w530) -> (x-y=w533:dbl)
          n311 = Split 1D Array(array=w526, index=w533) -> (first subarray=w527:sgl[])  [unwired: 1 out]
          n312 = Build Array (concatenate)(w528, w527) -> (w529:sgl[])
          n313 = Array Max & Min(array=w529) -> (max value=w537:sgl, min value=w536:sgl)  [unwired: 2 out]
          n314 = Subtract(x=w537, y=w536) -> (x-y=w539:sgl)
          n315 = Less?(x=w539, y=w540) -> (x < y?=w538:bool)
          n316 = Select(t=w540, s=w538, f=w539) -> (s? t:f=w541:sgl)
          n317 = Select(t=w534, s=w538, f=w537) -> (s? t:f=w543:sgl)
          n318 = Select(t=w535, s=w538, f=w536) -> (s? t:f=w542:sgl)
        }
        n319 = Complex To Re/Im(x + iy=w507) -> (x=w506:dbl[])  [unwired: 1 out]
        n320 = Initialize Array(w514, w513) -> (w510:sgl[])
        n321 = Initialize Array(w515, w513) -> (w509:sgl[])
        n322 = Build Array(w511, w506, w510, w509) -> (w508:dbl[][])
      }
      frame "Fk" {
        n323 = Unbundle By Name(w556) -> ("Engranometro.Cant. Dientes x pieza"=w549:i32)
        n324 = Array Size(array=w555) -> (size(s)=w552:i32)
        n325 = call-poly <vilib>:"FFT.vi"("FFT size"=w552, "X"=w555) -> ("FFT {X}"=w571:cdb[])  [unwired: 8 in, 1 out]
        n326 = Increment(x=w549) -> (x+1=w548:i32)
        n327 = Split 1D Array(array=w571, index=w548) -> (first subarray=w562:cdb[], second subarray=w569:cdb[])
        n328 = Array Size(array=w562) -> (size(s)=w564:i32)
        n329 = Subtract(x=w564, y=3) -> (x-y=w561:i32)
        n330 = Split 1D Array(array=w562, index=w561) -> (first subarray=w559:cdb[], second subarray=w558:cdb[])
        n331 = Split 1D Array(array=w569, index=2) -> (first subarray=w565:cdb[], second subarray=w567:cdb[])
        n332 = Multiply(x=cdb 0.0+0.0i, y=w559) -> (x*y=w557:cdb[])
        n333 = Multiply(x=w567, y=cdb 0.0+0.0i) -> (x*y=w566:cdb[])
        n334 = Build Array (concatenate)(w557, w558, w565, w566) -> (w546:cdb[])
        n335 = Multiply(x=2.0, y=w546) -> (x*y=w545:cdb[])
        n336 = call-poly <vilib>:"Inverse FFT.vi"("FFT {X}"=w545) -> ("X"=w551:cdb[])  [unwired: 9 in, 1 out]
        n337 = Complex To Re/Im(x + iy=w551) -> (x=w550:dbl[])  [unwired: 1 out]
        n338 = Array Max & Min(array=w550) -> (max value=w554:dbl, min value=w553:dbl)  [unwired: 2 out]
        n339 = Initialize Array(w554, w552) -> (w574:dbl[])
        n340 = Initialize Array(w553, w552) -> (w572:dbl[])
        n341 = Build Array(w555, w550, w574, w572) -> (w573:dbl[][])
      }
    }
    "Curva de Engranes" <- w250
  }
  n342 = call "MathLoop.vi"("CORE"=w10, "error in (no error)"=w11, "Solve notifier"=w7, "MATH"=w8, "ACQ Data Queue"=w9) -> ("error out"=w12:errorcluster)  [unwired: 6 in]
  n343 = Set Occurrence(w27) -> ()
  n344 = Merge Errors(w35, w17, w12) -> (w36:errorcluster)
  n345 = call "Destroy All Data Queues.vi"("Error In"=w36, "WINFAS 2 Data Queue.lvlib:All Data Queues Cluster"=w9) -> ("Error Out"=w42:errorcluster)  [unwired: 9 in]
  n346 = call "Destroy All Message Queues.vi"("error in (no error)"=w42, "Message Queues Out"=w33) -> ("error out"=w38:errorcluster)  [unwired: 9 in]
  n347 = Release Notifier(notifier=w7, error in (no error)=w38) -> (error out=w23:errorcluster)  [unwired: 1 in, 2 out]
  n348 = property class="App"(error in=w23) -> ("App.Kind"=w25:T7)  [unwired: 1 in, 2 out]
  n349 = case shown="\"Run Time System\"" w25 {
    tunnel: [TRUE FALSE TRUE] -> w24
    tunnel: [w622 w636 w642] -> _
    frame "invalid app kind", Default {
      n350 = property class="VI"() -> (error out=w623:errorcluster, "Panel"=w633:refnum<vi>)  [unwired: 2 in, 1 out]
      n351 = property class="Pnl"(reference=w633, error in=w623) -> (error out=w624:errorcluster, "AllObjs[]"=w632:refnum<vi>[])  [unwired: 1 out]
      n352 = control-ref of="This VI"() -> (w630:refnum<vi>)
      n353 = Close Reference(reference=w632, error in (no error)=w624) -> (error out=w629:errorcluster)
      n354 = invoke class="VI" method="FP.Close"(reference=w630, error in=w629) -> (reference out=w628:refnum<vi>, error out=w627:errorcluster)  [unwired: 1 in, 1 out]
      n355 = invoke class="VI" method="Abort VI"(reference=w628, error in=w627) -> (reference out=w625:refnum<vi>, error out=w626:errorcluster)  [unwired: 1 in, 1 out]
      n356 = control-ref of="This Application"() -> (w635:refnum<vi>)
      n357 = Close Reference(reference=w625, error in (no error)=w626) -> (error out=w634:errorcluster)
      n358 = Close Reference(reference=w635, error in (no error)=w634) -> (error out=w622:errorcluster)
    }
    frame "Development System" {
      n359 = property class="VI"() -> (error out=w637:errorcluster, "Panel"=w641:refnum<vi>)  [unwired: 2 in, 1 out]
      n360 = property class="Pnl"(reference=w641, error in=w637) -> (error out=w638:errorcluster, "AllObjs[]"=w640:refnum<vi>[])  [unwired: 1 out]
      n361 = Close Reference(reference=w640, error in (no error)=w638) -> (error out=w636:errorcluster)
    }
    frame "Run Time System" {
      n362 = property class="VI"() -> (error out=w643:errorcluster, "Panel"=w653:refnum<vi>)  [unwired: 2 in, 1 out]
      n363 = property class="Pnl"(reference=w653, error in=w643) -> (error out=w644:errorcluster, "AllObjs[]"=w652:refnum<vi>[])  [unwired: 1 out]
      n364 = control-ref of="This VI"() -> (w650:refnum<vi>)
      n365 = Close Reference(reference=w652, error in (no error)=w644) -> (error out=w649:errorcluster)
      n366 = invoke class="VI" method="FP.Close"(reference=w650, error in=w649) -> (reference out=w648:refnum<vi>, error out=w647:errorcluster)  [unwired: 1 in, 1 out]
      n367 = invoke class="VI" method="Abort VI"(reference=w648, error in=w647) -> (reference out=w645:refnum<vi>, error out=w646:errorcluster)  [unwired: 1 in, 1 out]
      n368 = control-ref of="This Application"() -> (w655:refnum<vi>)
      n369 = Close Reference(reference=w645, error in (no error)=w646) -> (error out=w654:errorcluster)
      n370 = Close Reference(reference=w655, error in (no error)=w654) -> (error out=w642:errorcluster)
    }
  }
  n371 = Quit LabVIEW(quit? (T)=w24) -> ()
